vi "Main.vi"() -> ()   [LabVIEW 2020]
uses:
  <vilib>/userDefined/High Color/IMAQdx.ctl
  <vilib>/vision/driver/NI_Vision_Acquisition_Software.lvlib
panel:
  out "Status":bool
  in  "Off/On":bool caption="Start/Stop Vision"
  out "IMAQ Err":errorcluster
  out "Live view":T1(plugin-control)
  out "Python Error Out":errorcluster
  out "Camera Status":errorcluster
  in  "Exit program":bool
  in  "Camera Device":T2="cam0"
  # "Vision control panel"
  # "Camera configuration"
  # "Error section"
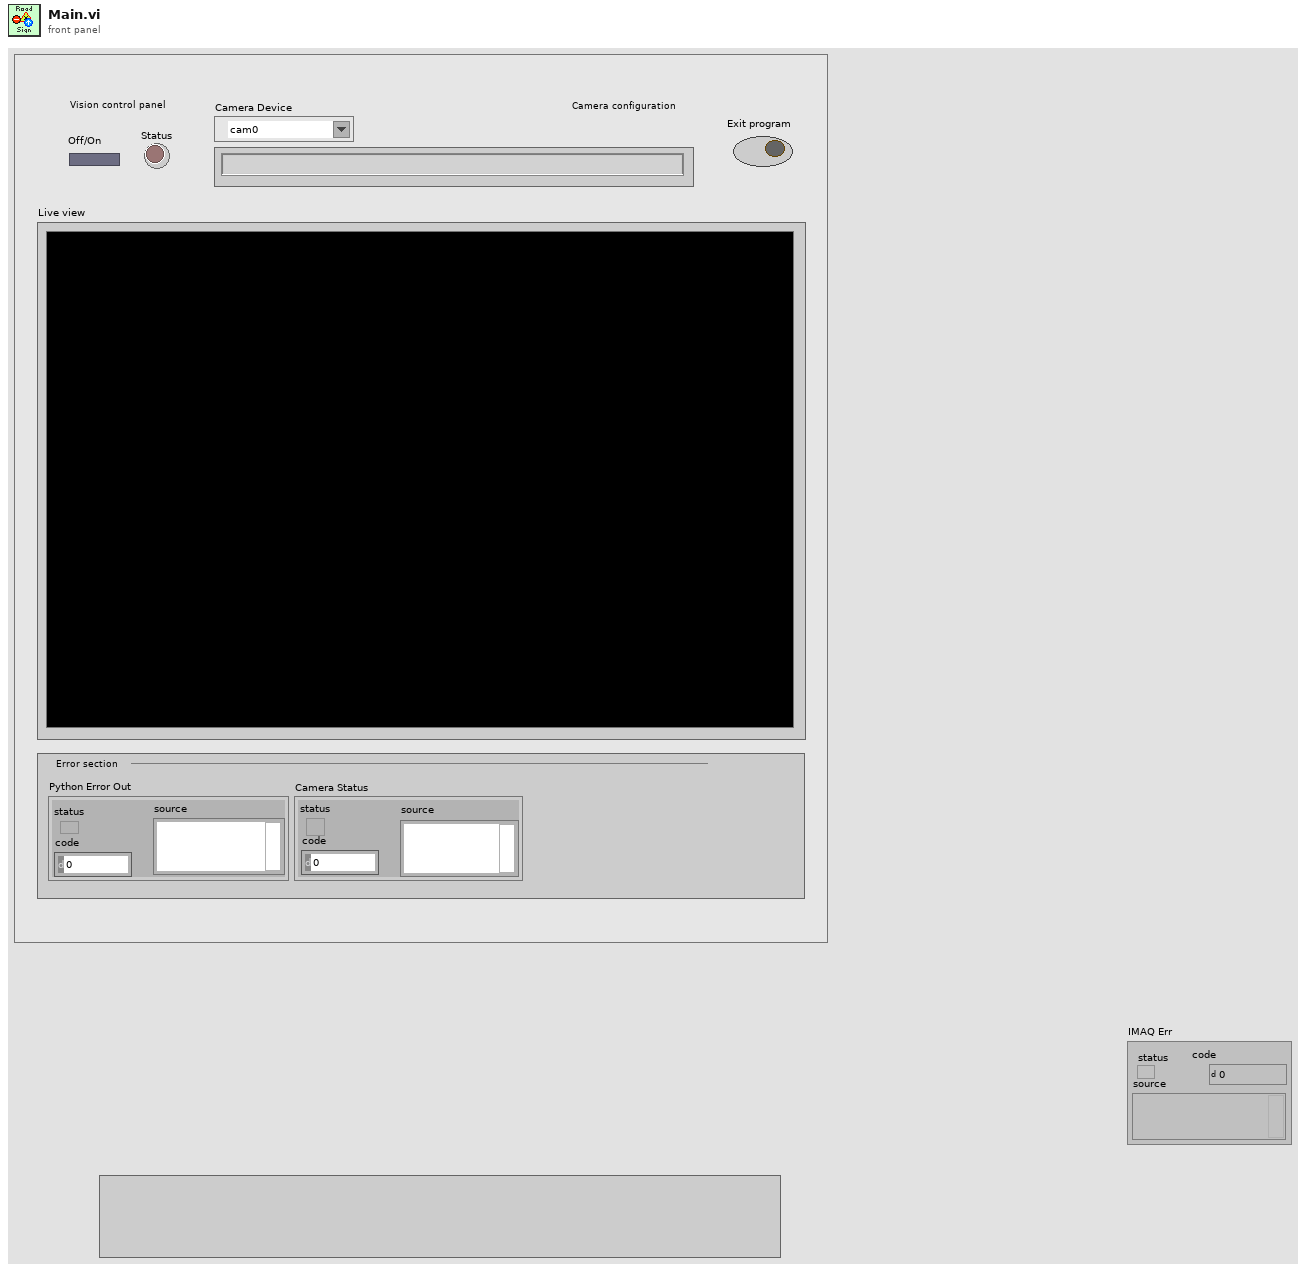
[diagram p1: front panel]
types:
  T1 = typedef "IMAQ Image.ctl" = refnum<image>
  T2 = typedef "IMAQdx.ctl" = refnum<k21>
  T3 = enum32{"Invalid", "Standard", "Closed", "Hidden", "Minimized", "Maximized"}
  T4 = enum32{"invalid app kind", "Development System", "Run Time System", "Student Edition", "Embedded LabVIEW", "Evaluation", "Custom"}
  T5 = cluster{"Core":cluster{"Current VI Reference":refnum<vi>, "Close Panel on Exit?":bool}, "Camera Device":T2}
  T6 = cluster{"Current VI Reference":refnum<vi>, "Close Panel on Exit?":bool}
  T7 = typedef "Image Type" = u32
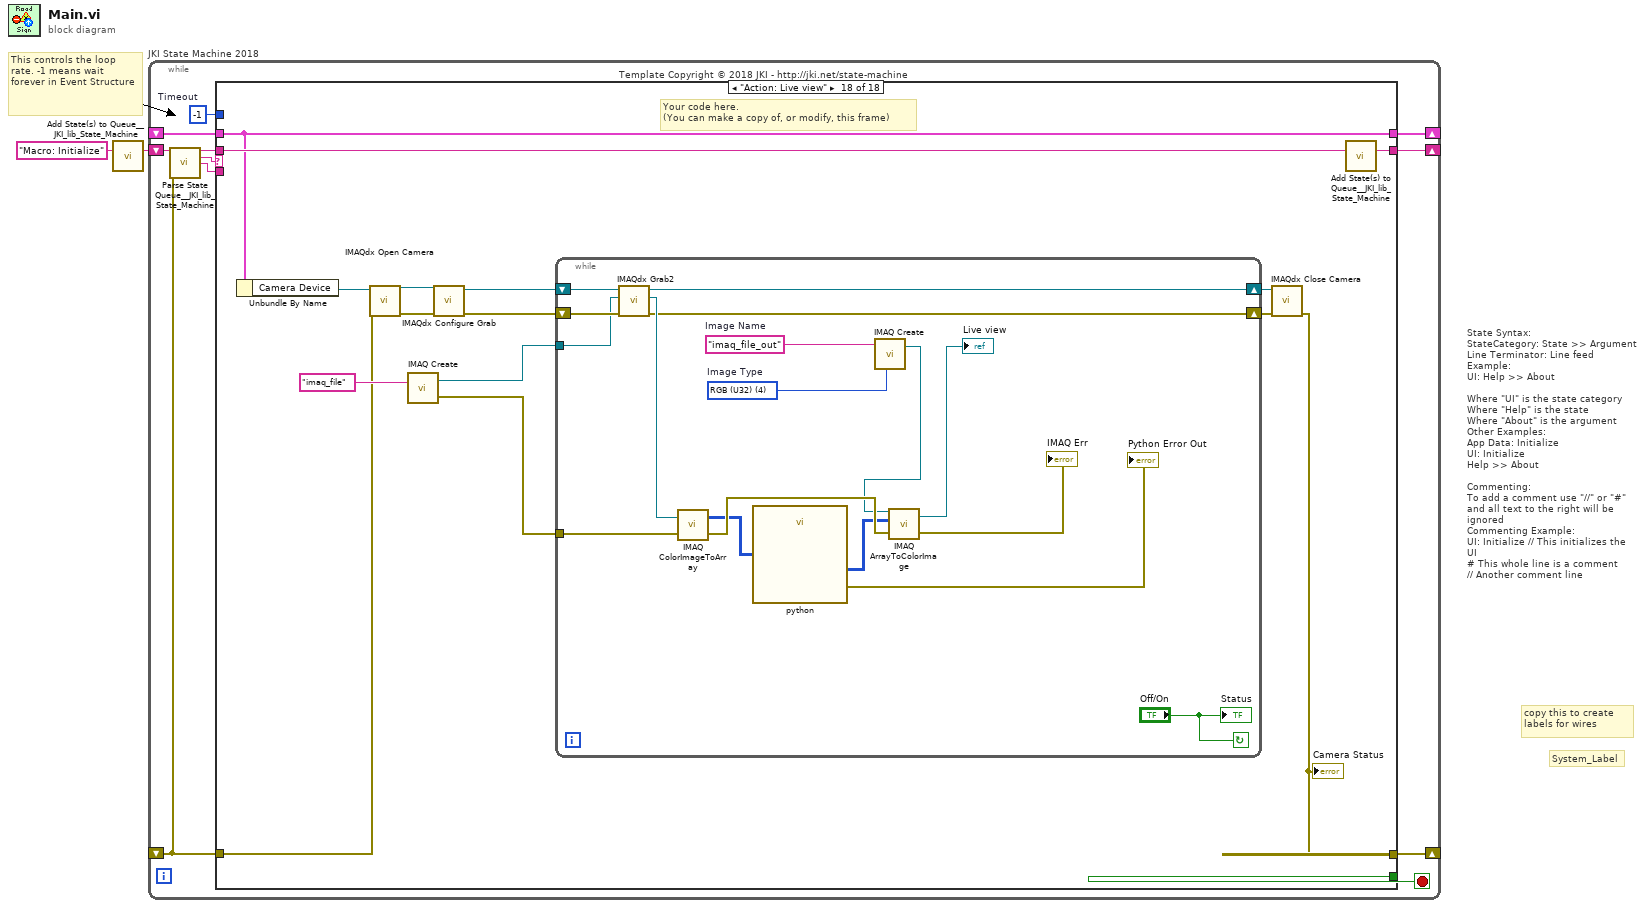
[diagram p0: block diagram]
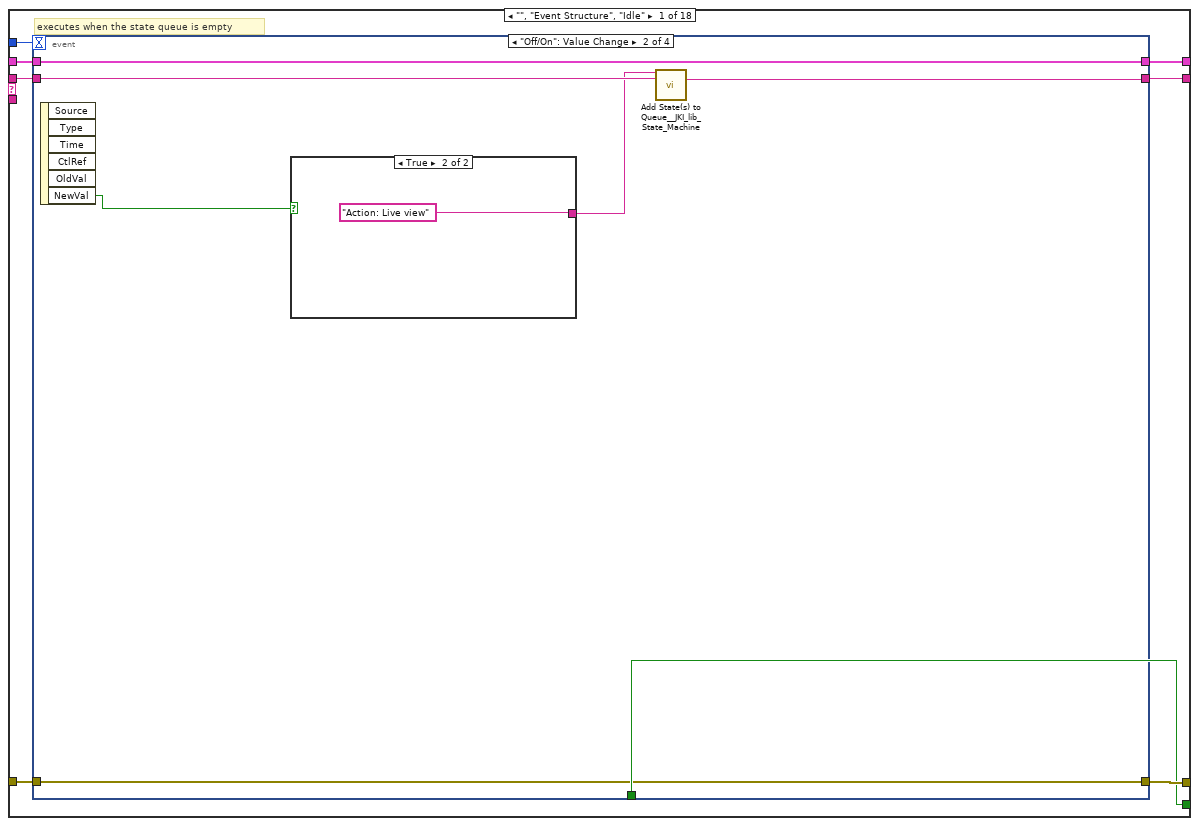
[diagram p2: hidden frame]
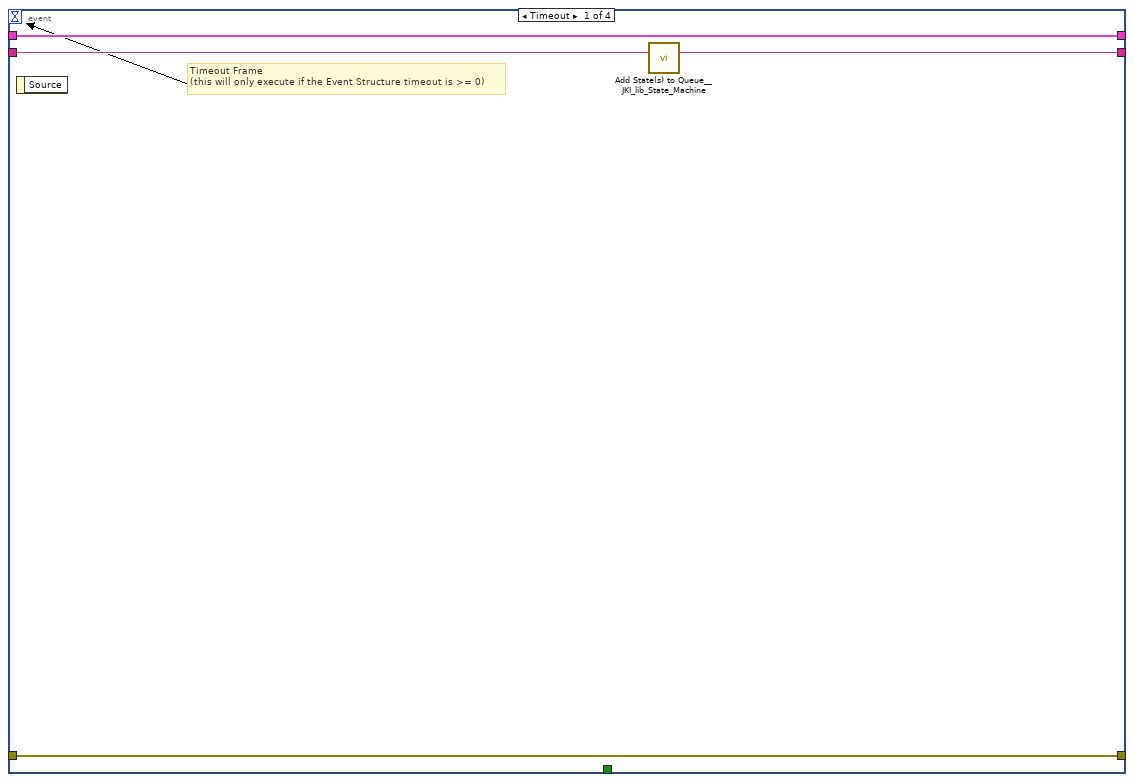
[diagram p3: hidden frame]
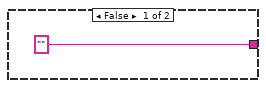
[diagram p4: hidden frame]
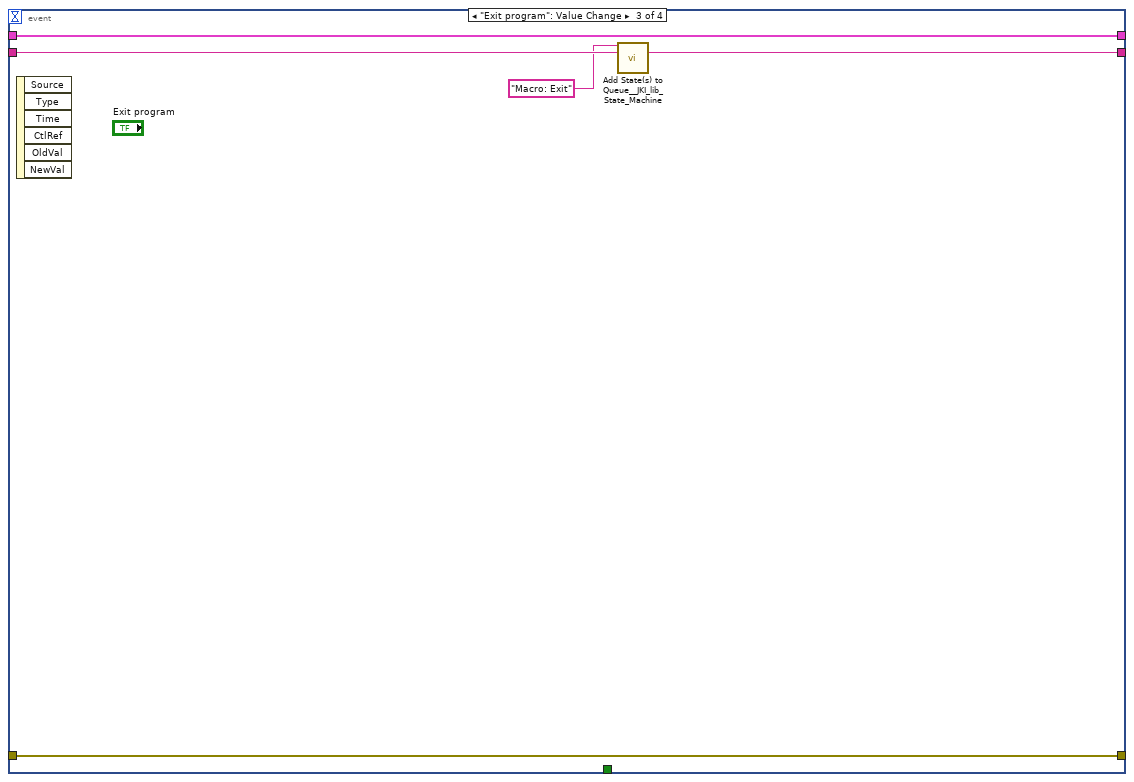
[diagram p5: hidden frame]
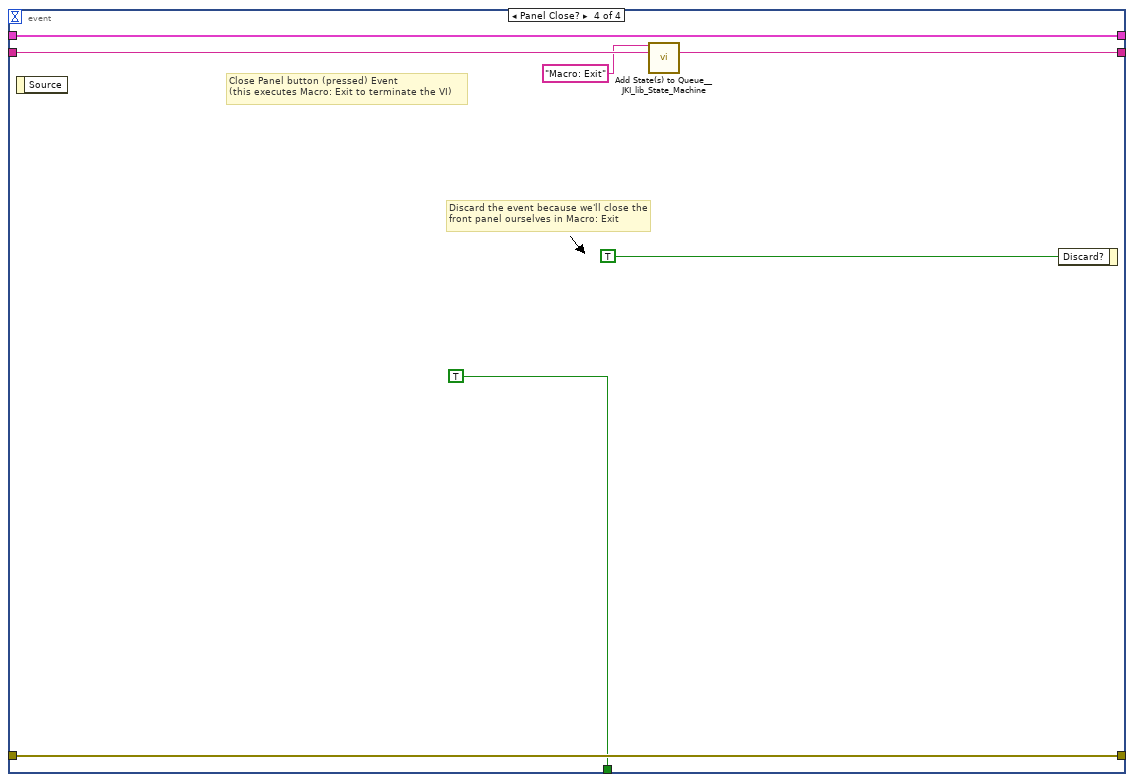
[diagram p6: hidden frame]
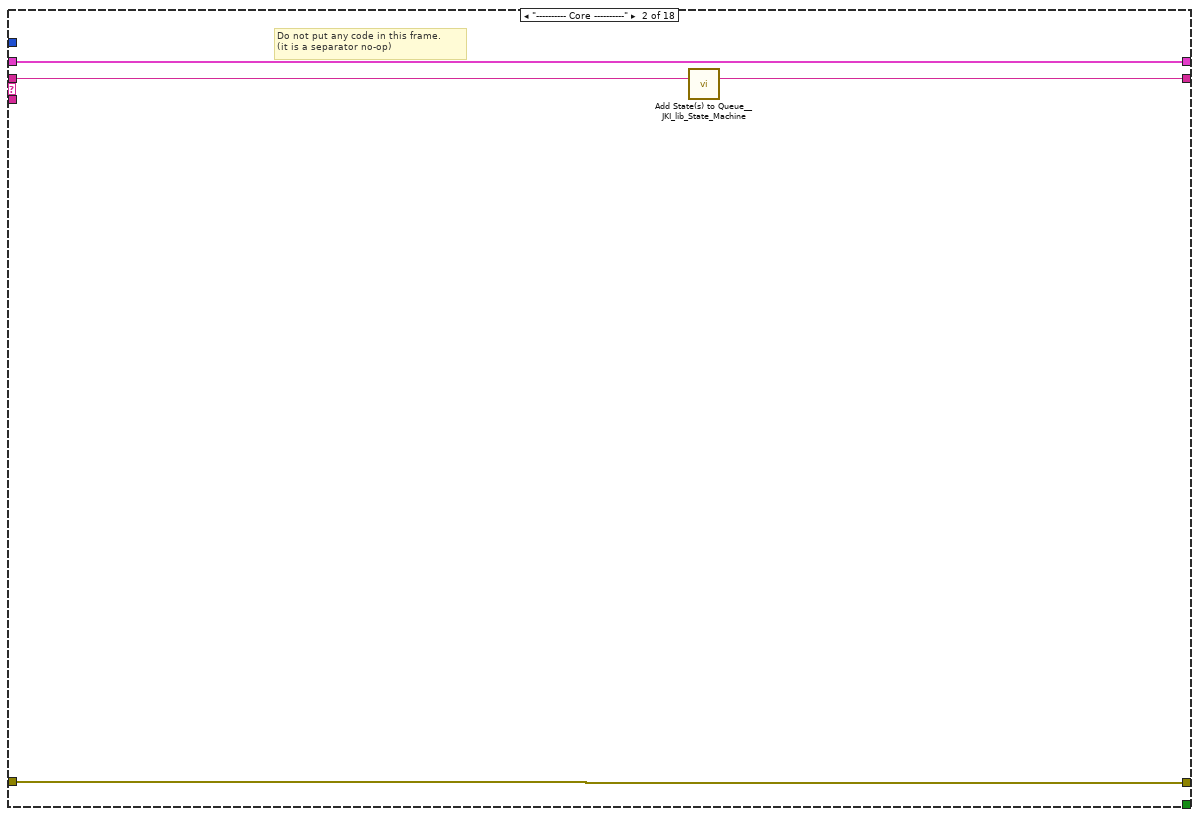
[diagram p7: hidden frame]
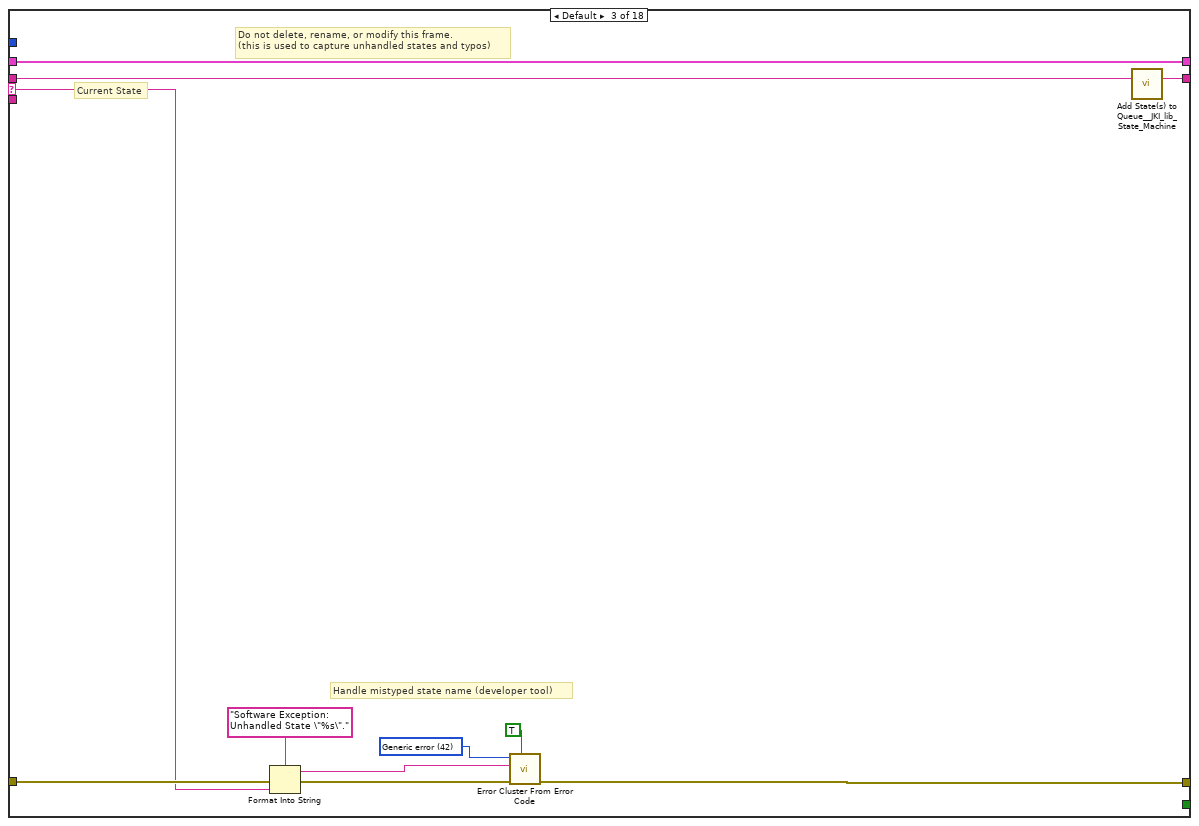
[diagram p8: hidden frame]
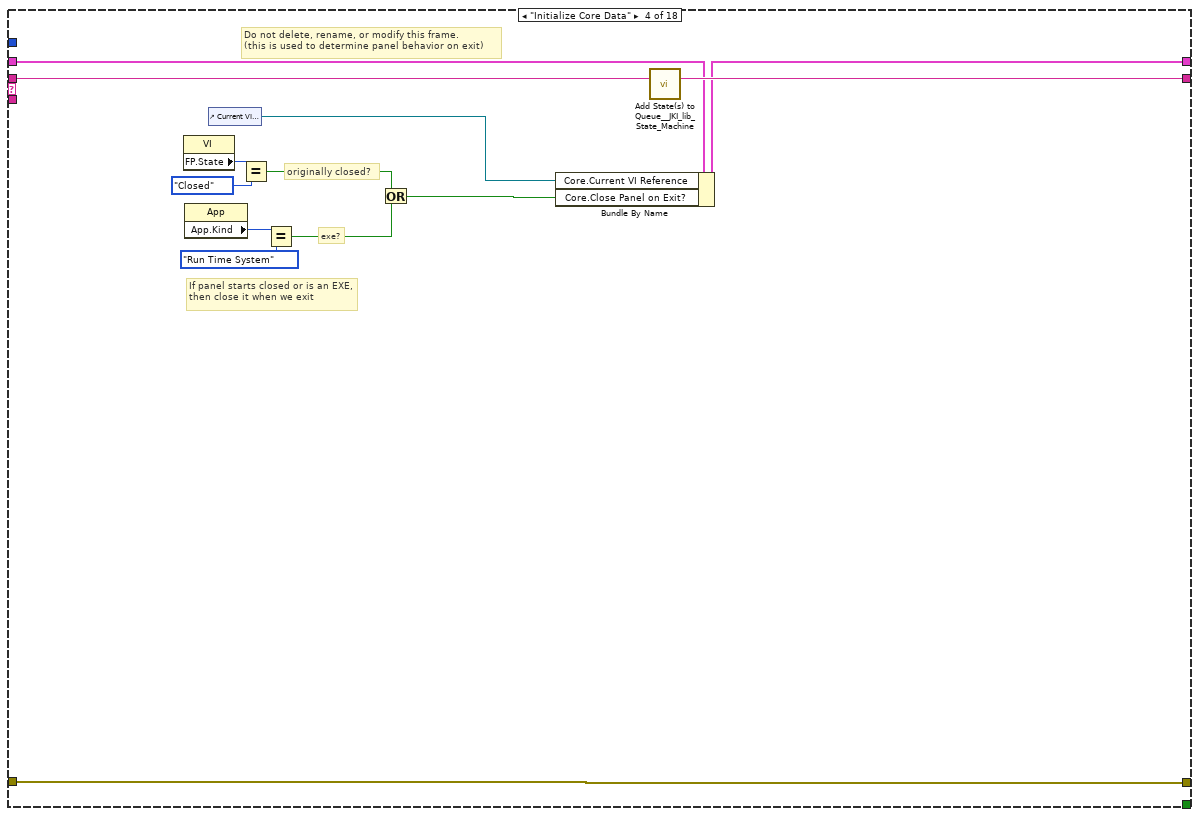
[diagram p9: hidden frame]
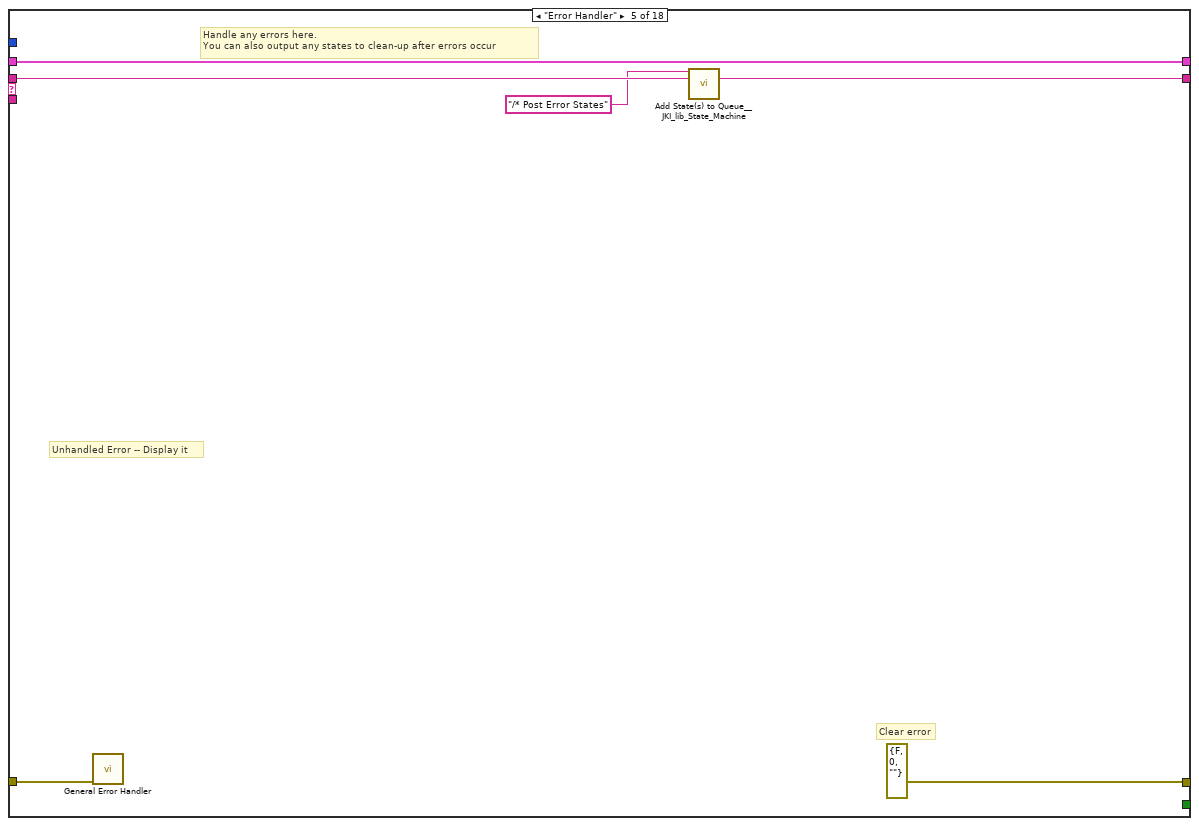
[diagram p10: hidden frame]
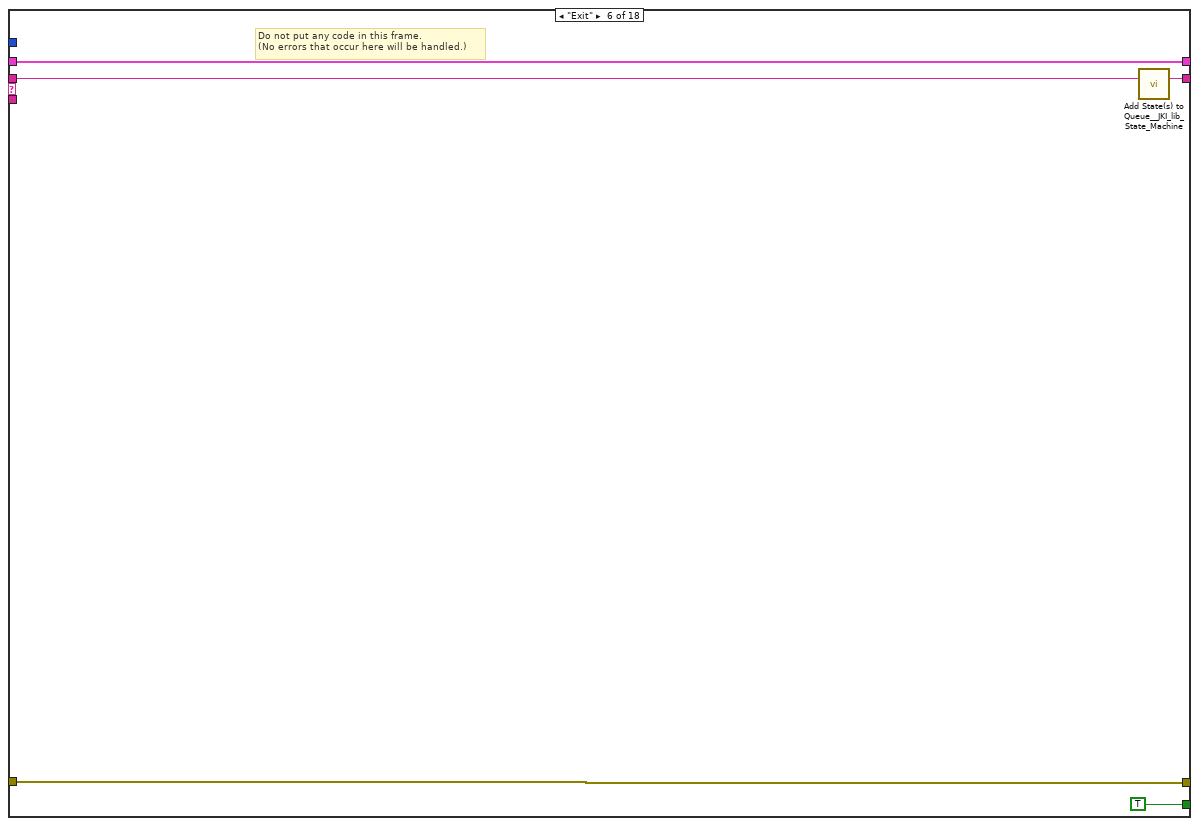
[diagram p11: hidden frame]
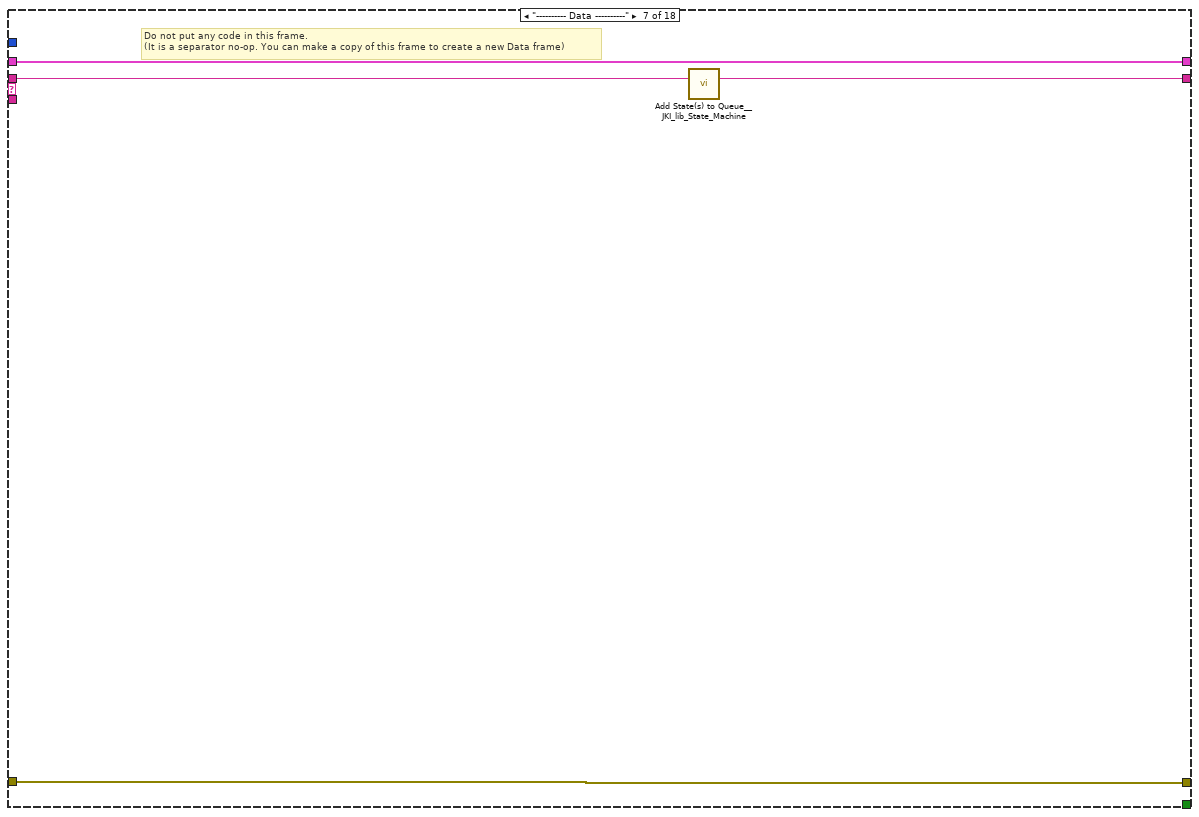
[diagram p12: hidden frame]
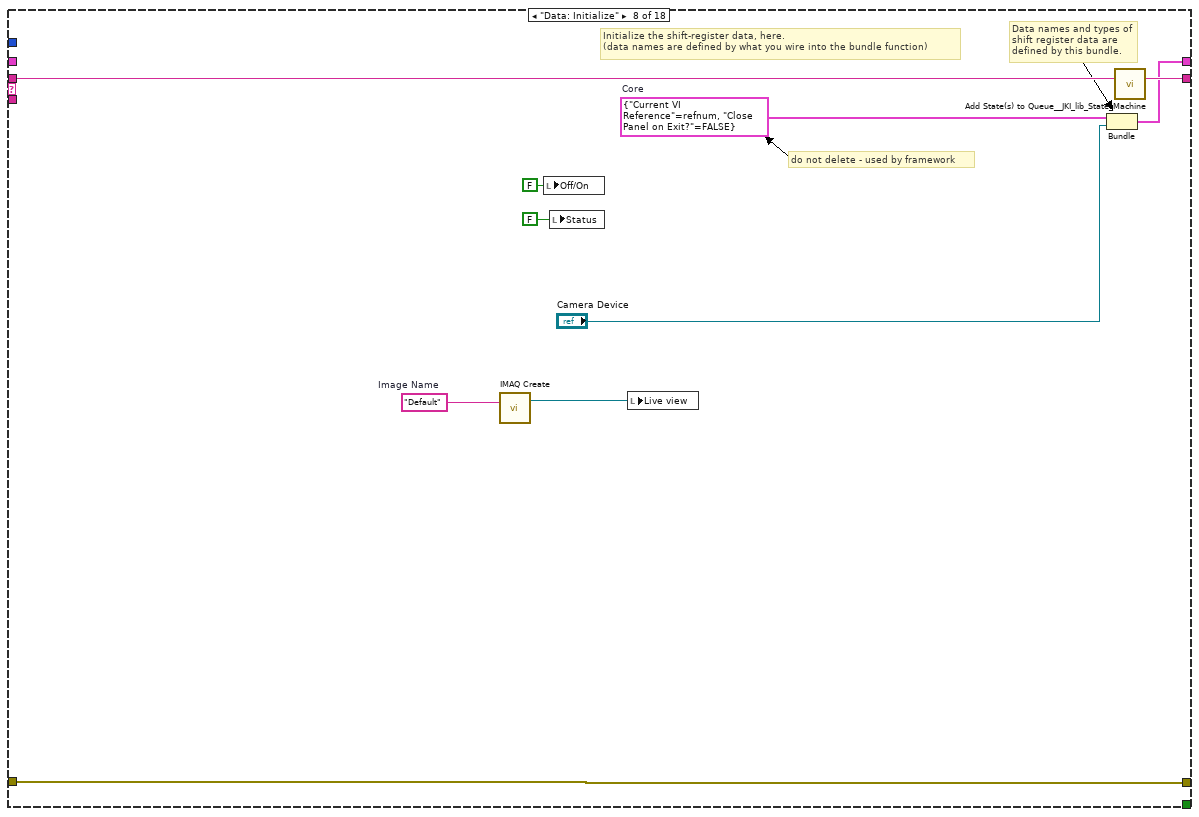
[diagram p13: hidden frame]
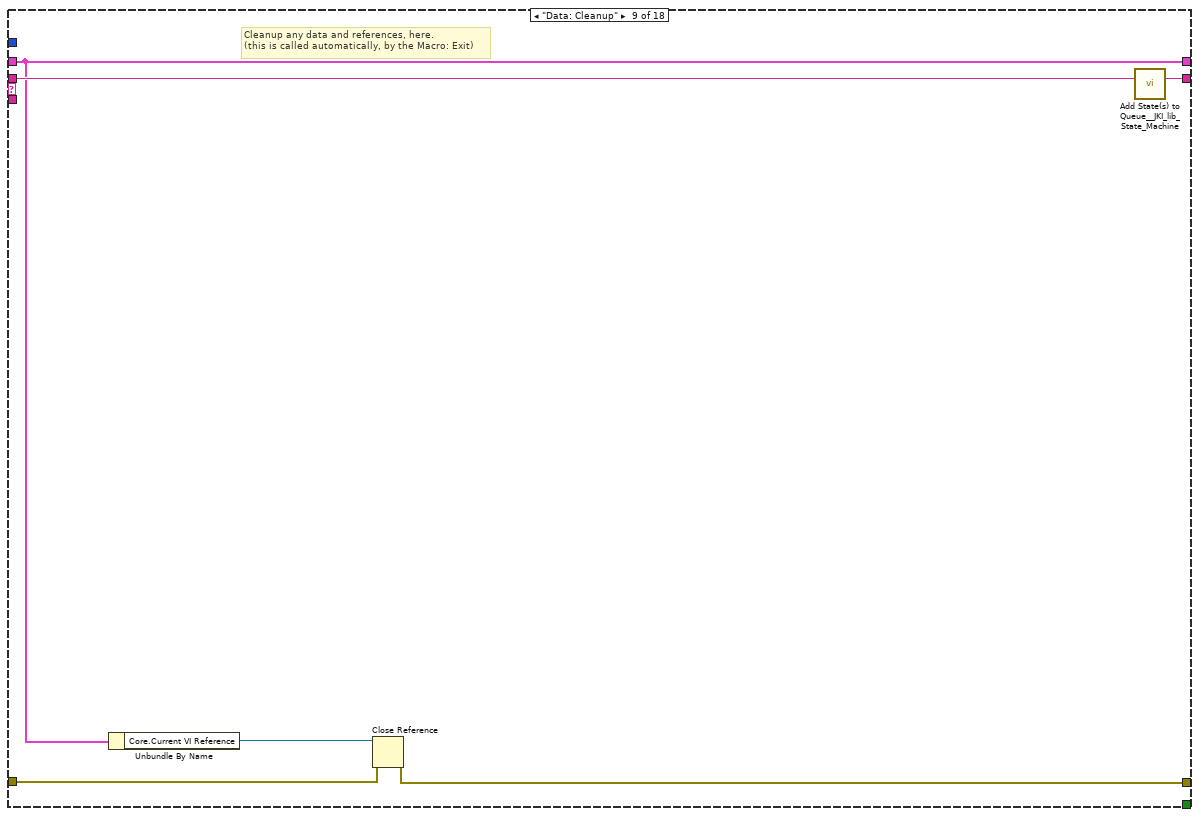
[diagram p14: hidden frame]
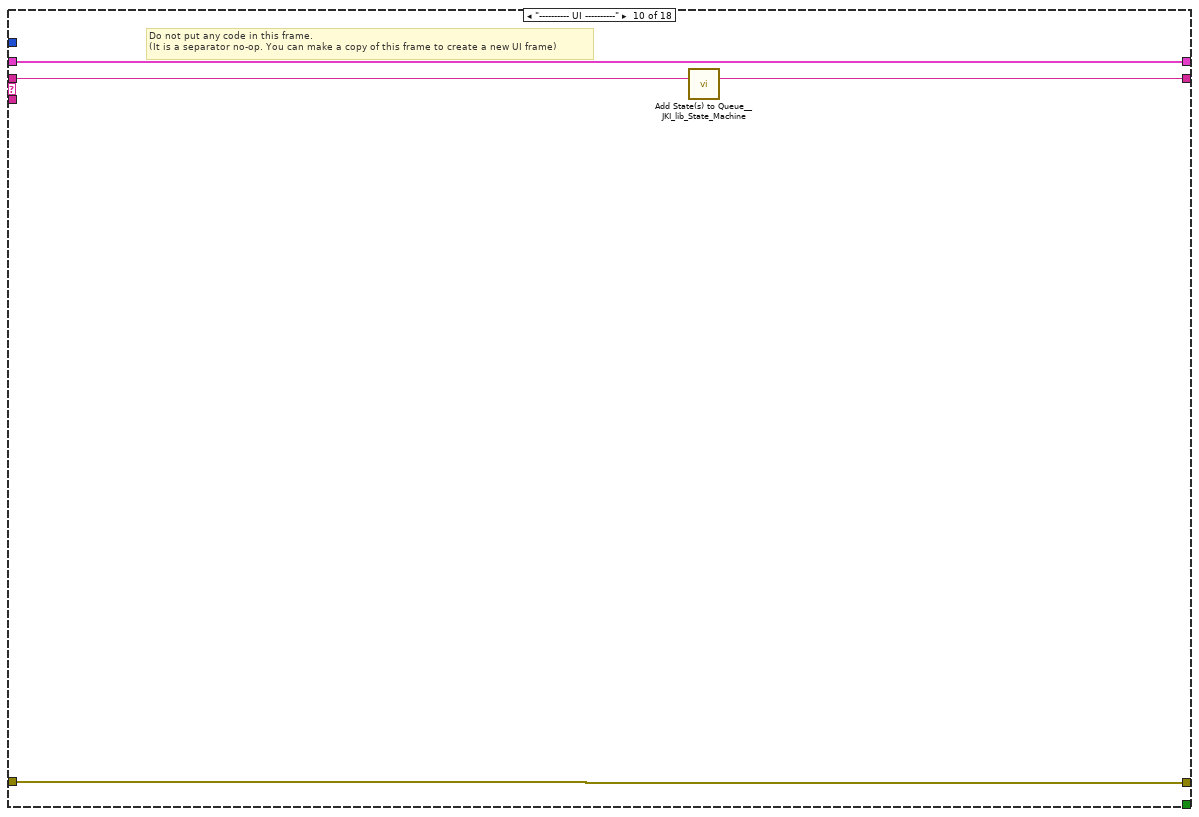
[diagram p15: hidden frame]
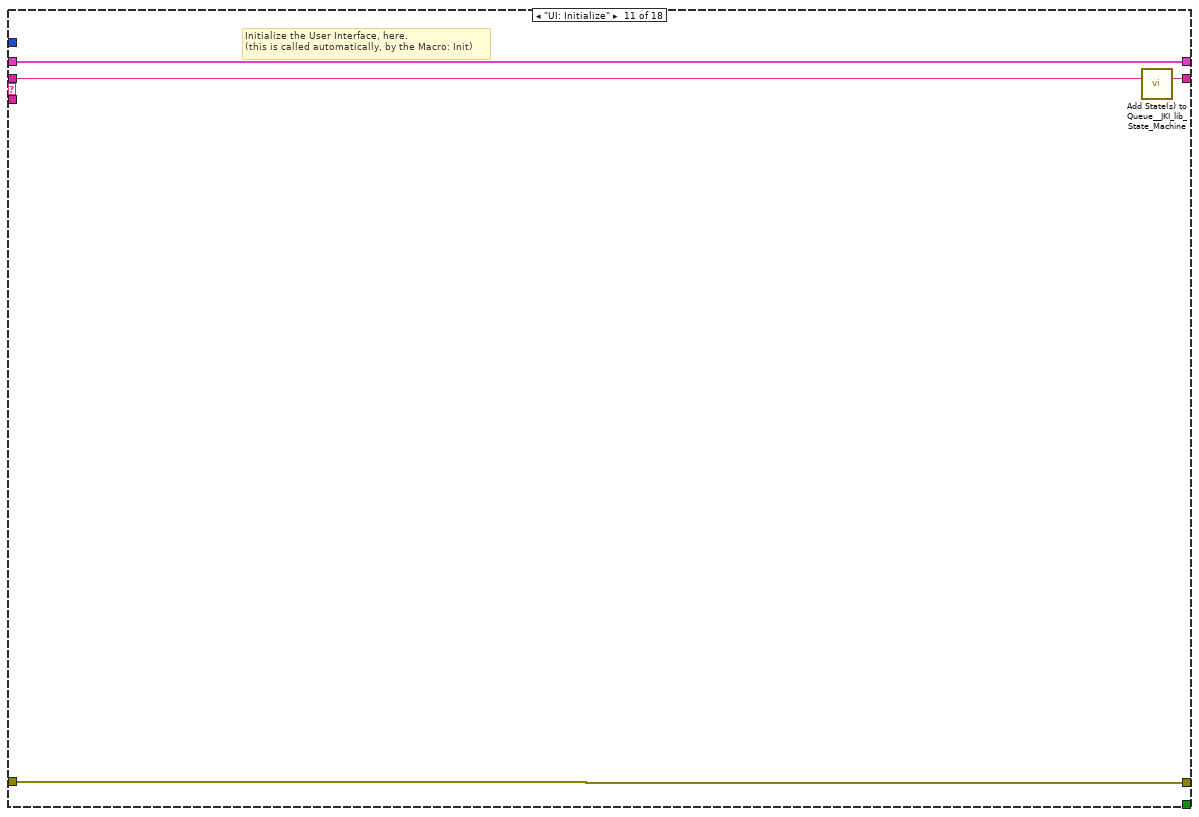
[diagram p16: hidden frame]
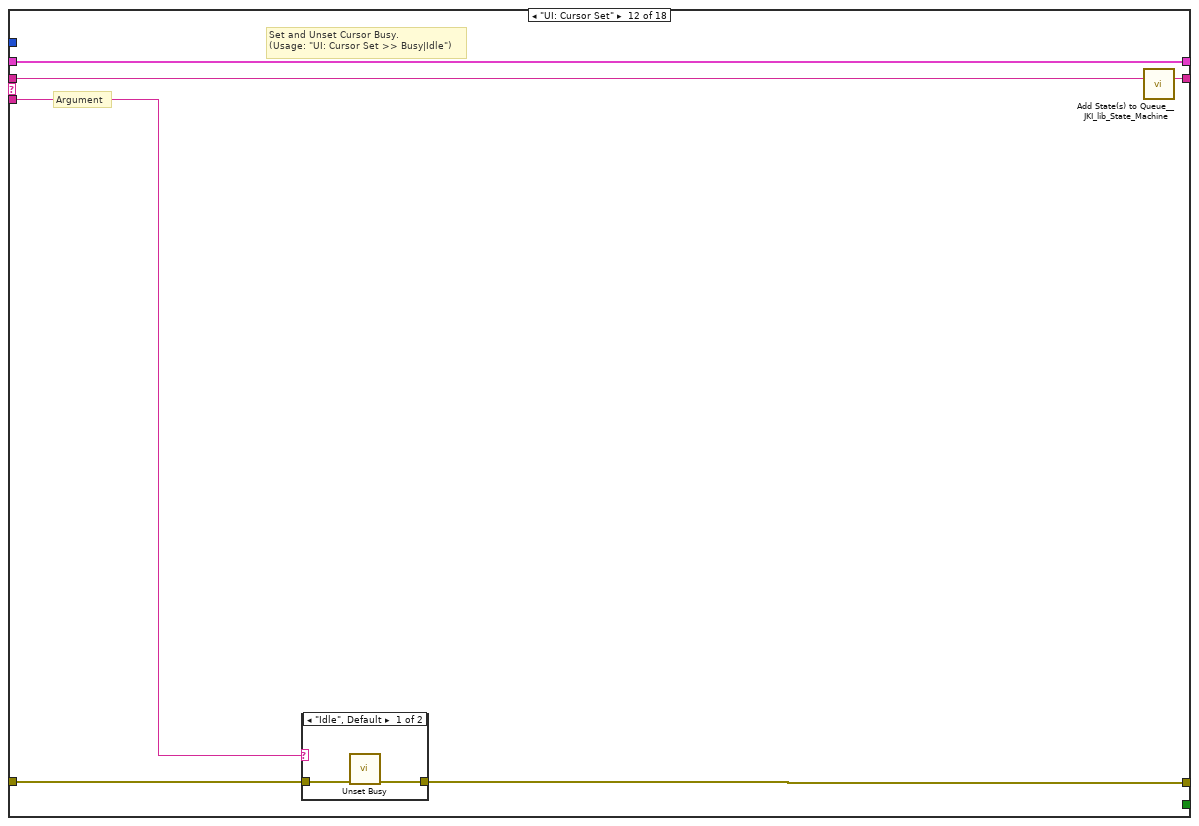
[diagram p17: hidden frame]
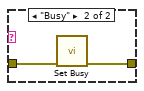
[diagram p18: hidden frame]
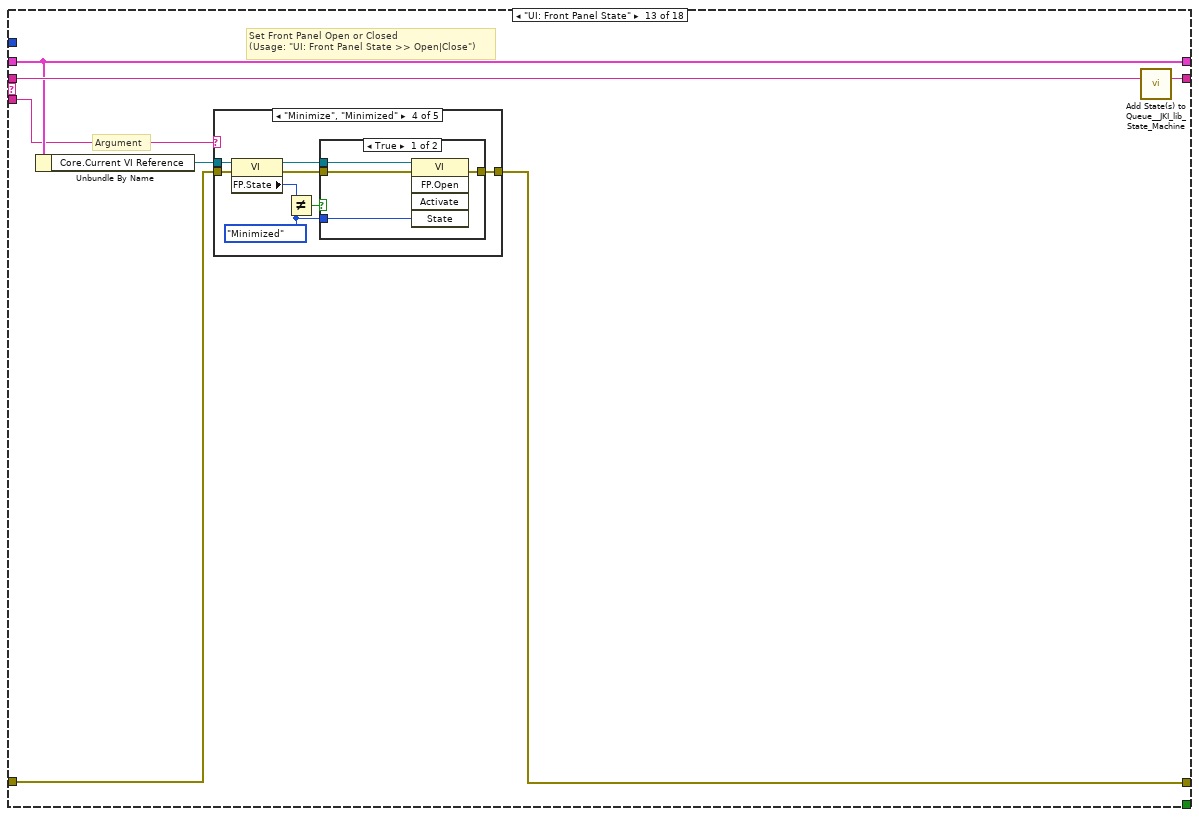
[diagram p19: hidden frame]
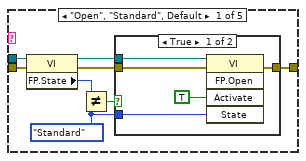
[diagram p20: hidden frame]
diagram:
  # "State Syntax:\nStateCategory: State >> Argument\nLine Terminator: Line feed\nExample:\nUI: Help >> About\n\nWhere \"UI\" is the state category\nWhere \"Help\" is the state\nWhere \"About\" is the argument\nOther Examples:\nApp Data: Initialize\nUI: Initialize\nHelp >> About\n\nCommenting:\nTo add a comment use \"//\" or \"#\" and all text to the right will be ignored\nCommenting Example:\nUI: Initialize // This initializes the UI\n# This whole line is a comment\n// Another comment line"
  # "copy this to create labels for wires"
  # "This controls the loop rate. -1 means wait forever in Event Structure"
  # "System_Label"
  n1 = call <vilib>:"Add State(s) to Queue__JKI_lib_State_Machine.vi"("State(s) in (\"\")"="Macro: Initialize") -> ("States Out"=w2:string)  [unwired: 14 in]
  n2 = while "JKI State Machine 2018" {
    shift-right: [w6] -> _
    shift-left: _ -> [w5]
    shift-right: [w9] -> _
    shift-left: _ -> [w3]
    shift-right: [w8] -> _
    shift-left: w2 -> [w10]
    stop <- w7 stop-if-true
    w4 = -1  # Timeout
    # "Template Copyright © 2018 JKI - http://jki.net/state-machine"
    n3 = call <vilib>:"Parse State Queue__JKI_lib_State_Machine.vi"("State Queue"=w10, "Error In (no error)"=w3) -> ("Remaining States"=w12:string, "Current State"=w13:string, "Arguments"=w11:string)  [unwired: 11 in]
    n4 = case shown="\"Action: Live view\"" w13 {
      selector: w13 -> [_ _ w50 _ _ _ _ _ _ _ _ _ _ _ _ _ _ _]
      tunnel: w12 -> [w21 w49 w54 w73 w79 w84 w88 w98 w104 w108 w112 w118 w129 w198 w203 w213 w217 w232]
      tunnel: w11 -> [_ _ _ _ _ _ _ _ _ _ _ w113 w123 _ _ _ _ _]
      tunnel: w5 -> [w19 w46 w52 w66 w76 w82 w85 _ w99 w105 w110 w116 w125 w195 w200 w210 w214 w228]
      tunnel: [w18 w47 w56 w70 errorcluster {"status"=FALSE, "code"=0, "source"=""} ("error out") w81 w86 w95 w100 w106 w109 w114 w126 w196 w201 w211 w215 w224] -> w9
      tunnel: w3 -> [w17 w47 w55 w70 w75 w81 w86 w95 w101 w106 w109 w115 w127 w196 w201 w211 w215 w225]
      tunnel: [w20 w48 w53 w72 w78 w83 w87 w97 w103 w107 w111 w117 w128 w197 w202 w212 w216 w231] -> w8
      tunnel: [w14 _ _ _ _ TRUE _ _ _ _ _ _ _ _ _ _ _ _] -> w7
      tunnel: [w16 w46 w52 w71 w76 w82 w85 w96 w99 w105 w110 w116 w125 w195 w200 w210 w214 w228] -> w6
      tunnel: w4 -> [w15 _ _ _ _ _ _ _ _ _ _ _ _ _ _ _ _ _]
      frame "", "Event Structure", "Idle" {
        # "executes when the state queue is empty"
        n5 = event shown="[1] \"Off/On\": Value Change" {
          selector: _ -> [_ _ _ _]
          dyn-events: _ -> [_ _ _ _]
          timeout: w15 -> [_ _ _ _]
          tunnel: w21 -> [w25 w28 w36 w45]
          tunnel: [w24 w29 w37 w44] -> w20
          tunnel: w19 -> [w22 w31 w38 w42]
          tunnel: [w23 w30 w34 w43] -> w18
          tunnel: w17 -> [w23 w30 w34 w43]
          tunnel: [w22 w31 w38 w42] -> w16
          tunnel: [_ _ _ TRUE] -> w14
          event Timeout {
            # "Timeout Frame\n(this will only execute if the Event Structure timeout is >= 0)"
            n6 = event-data() -> ()  [unwired: 1 in, 1 out]
            n7 = call <vilib>:"Add State(s) to Queue__JKI_lib_State_Machine.vi"("State(s) in (\"\")"=w25) -> ("States Out"=w24:string)  [unwired: 14 in]
          }
          event "Off/On": Value Change {
            n8 = event-data() -> ("NewVal"=w26:bool)  [unwired: 1 in, 5 out]
            n9 = case shown="True" w26 {
              tunnel: ["" "Action: Live view" ("State(s) in Front (\"\")")] -> w27
              frame False {
              }
              frame True {
              }
            }
            n10 = call <vilib>:"Add State(s) to Queue__JKI_lib_State_Machine.vi"("State(s) in Front (\"\")"=w27, "State(s) in (\"\")"=w28) -> ("States Out"=w29:string)  [unwired: 13 in]
          }
          event "Exit program": Value Change {
            n11 = event-data() -> ()  [unwired: 1 in, 6 out]
            n12 = call <vilib>:"Add State(s) to Queue__JKI_lib_State_Machine.vi"("State(s) in Front (\"\")"="Macro: Exit" ("State(s) in Front (\"\")"), "State(s) in (\"\")"=w36) -> ("States Out"=w37:string)  [unwired: 13 in]
          }
          event Panel Close? {
            # "Discard the event because we'll close the front panel ourselves in Macro: Exit"
            # "Close Panel button (pressed) Event\n(this executes Macro: Exit to terminate the VI)"
            n13 = event-data() -> ()  [unwired: 1 in, 1 out]
            n14 = call <vilib>:"Add State(s) to Queue__JKI_lib_State_Machine.vi"("State(s) in Front (\"\")"="Macro: Exit", "State(s) in (\"\")"=w45) -> ("States Out"=w44:string)  [unwired: 13 in]
            n15 = event-data("Discard?"=TRUE) -> ()  [unwired: 1 in, 1 out]
          }
        }
      }
      frame "---------- Core ----------" {
        # "Do not put any code in this frame.\n(it is a separator no-op)"
        n16 = call <vilib>:"Add State(s) to Queue__JKI_lib_State_Machine.vi"("State(s) in (\"\")"=w49) -> ("States Out"=w48:string)  [unwired: 14 in]
      }
      frame Default {
        w59 = 42 items=["No error", "Argument error", "Memory is full", "Out of zone", "End of file", "File already open", "Generic file I/O error", "File not found", "File permission error", "Disk is full", "Duplicate path", "Too many files open", "System feature not enabled", "Resource file not found", "Cannot add resource", "Resource not found", "Image not found", "Image memory error", "Pen does not exist", "Config type invalid", "Config token not found", "Config parse error", "Config memory error", "Bad external code format", "Bad external code offset", "External code not present", "Null window", "Destroy window error", "Null menu", "Print aborted", "Bad print record", "Print driver error", "Windows error during printing", "Memory error during printing", "Print dialog error", "Generic print error", "Invalid device refnum", "Device not found", "Device parameter error", "Device unit error", "Cannot open device", "Device call aborted", "Generic error", "Cancelled by user", "Object ID too low", "Object ID too high", "Object not in heap", "Unknown heap", "Unknown object (invalid DefProc)", "Unknown object (DefProc not in table)", "Message out of range", "Invalid (null) method", "Unknown message", "Manager call not supported", "Bad address", "Network operation in progress", "Network operation timed out", "Connection is busy", "Network attribute not supported", "Network error", "Address in use", "System out of memory", "Connection aborted", "Connection refused", "Not connected", "Already connected", "Connection closed", "Initialization error (interapplication manager)", "Bad occurrence", "Wait on unbound occurrence handler", "Occurrence queue overflow", "Datalog type conflict", "Unused", "Unrecognized type (interapplication manager)", "Memory corrupt", "Failed to make temporary DLL", "Old CIN version", "Drag socket not found", "Failed to load drop-object", "Failed to register OLE object", "Failed to release OLE object", "Format specifier type mismatch", "Unknown format specifier", "Too few format specifiers", "Too many format specifiers", "Scan failed", "Newer CIN version", "Error converting to variant", "Runtime menu error", "Password tampered", "Variant attribute not found", "Incompatible variant data type", "Event data is not available", "Event Store is not present", "Occurrence is not found", "Event Queue is not created", "Event info is not available", "Refnum passed is NULL", "Error retrieving Class GUID", "Error retrieving CoClass GUID", "Error retrieving TypeLib GUID.", "Bad built application magic bytes.", "Specific driver is different from the specific driver associated with the Logical Name.", "There is no session opened to the class driver.", "Max Error", "MAX - Error with config objects", "MAX - Error loading configuration", "MAX - Group not supported"]
        # "Current State"
        # "Do not delete, rename, or modify this frame.\n(this is used to capture unhandled states and typos)"
        # "Handle mistyped state name (developer tool)"
        n17 = Format Into String(format string="Software Exception: Unhandled State \"%s\"." ("message"), error in=w55, w50) -> (resulting string=w58:string, error out=w57:errorcluster)  [unwired: 1 in]
        n18 = call <vilib>:"Error Cluster From Error Code.vi"("show call chain? (False)"=TRUE, "error in (no error)"=w57, "error message (\"\")"=w58, "error code (0)"=w59) -> ("error out"=w56:errorcluster)  [unwired: 5 in]
        n19 = call <vilib>:"Add State(s) to Queue__JKI_lib_State_Machine.vi"("State(s) in (\"\")"=w54) -> ("States Out"=w53:string)  [unwired: 14 in]
      }
      frame "Initialize Core Data" {
        # "Do not delete, rename, or modify this frame.\n(this is used to determine panel behavior on exit)"
        # "originally closed?"
        # "exe?"
        # "If panel starts closed or is an EXE, then close it when we exit"
        n20 = property class="VI"() -> ("FP.State"=w63:T3)  [unwired: 2 in, 2 out]
        n21 = property class="App"() -> ("App.Kind"=w69:T4)  [unwired: 2 in, 2 out]
        n22 = control-ref of="Current VI Reference"() -> (w64:refnum<vi>)
        n23 = Equal?(x=w63, y=T3."Closed" ("Front Panel Window:State")) -> (x = y?=w61:bool)
        n24 = Equal?(x=w69, y=T4."Run Time System" ("Application:Kind")) -> (x = y?=w67:bool)
        n25 = Or(x=w61, y=w67) -> (x .or. y?=w65:bool)
        n26 = Bundle By Name(cluster=w66, "Core.Current VI Reference"=w64, "Core.Close Panel on Exit?"=w65) -> (w71:T5)
        n27 = call <vilib>:"Add State(s) to Queue__JKI_lib_State_Machine.vi"("State(s) in (\"\")"=w73) -> ("States Out"=w72:string)  [unwired: 14 in]
      }
      frame "Error Handler" {
        # "Unhandled Error -- Display it"
        # "Handle any errors here.\nYou can also output any states to clean-up after errors occur"
        # "Clear error"
        n28 = call <vilib>:"General Error Handler.vi"("error in (no error)"=w75) -> ()  [unwired: 10 in, 5 out]
        n29 = call <vilib>:"Add State(s) to Queue__JKI_lib_State_Machine.vi"("State(s) in Front (\"\")"="/* Post Error States", "State(s) in (\"\")"=w79) -> ("States Out"=w78:string)  [unwired: 13 in]
      }
      frame "Exit" {
        # "Do not put any code in this frame.\n(No errors that occur here will be handled.)"
        n30 = call <vilib>:"Add State(s) to Queue__JKI_lib_State_Machine.vi"("State(s) in (\"\")"=w84) -> ("States Out"=w83:string)  [unwired: 14 in]
      }
      frame "---------- Data ----------" {
        # "Do not put any code in this frame.\n(It is a separator no-op. You can make a copy of this frame to create a new Data frame)"
        n31 = call <vilib>:"Add State(s) to Queue__JKI_lib_State_Machine.vi"("State(s) in (\"\")"=w88) -> ("States Out"=w87:string)  [unwired: 14 in]
      }
      frame "Data: Initialize" {
        w90 = "Default"  # Image Name
        w94 = T6 {"Current VI Reference"=refnum, "Close Panel on Exit?"=FALSE}  # Core
        # "do not delete - used by framework"
        # "Data names and types of shift register data are defined by this bundle."
        # "Initialize the shift-register data, here.\n(data names are defined by what you wire into the bundle function)"
        n32 = call "IMAQ Create"("Image Name"=w90) -> ("New Image"=w89:T1)  [unwired: 4 in, 1 out]
        n33 = local write "Off/On"(FALSE ("Status")) -> ()
        n34 = local write "Status"(FALSE ("Off/On")) -> ()
        n35 = local write "Live view"(w89) -> ()
        n36 = Bundle("Core"=w94, "Camera Device"="Camera Device") -> (w96:T5)  [unwired: 1 in]
        n37 = call <vilib>:"Add State(s) to Queue__JKI_lib_State_Machine.vi"("State(s) in (\"\")"=w98) -> ("States Out"=w97:string)  [unwired: 14 in]
      }
      frame "Data: Cleanup" {
        # "Cleanup any data and references, here.\n(this is called automatically, by the Macro: Exit)"
        n38 = Unbundle By Name(w99) -> ("Core.Current VI Reference"=w102:refnum<vi>)
        n39 = Close Reference(reference=w102, error in (no error)=w101) -> (error out=w100:errorcluster)
        n40 = call <vilib>:"Add State(s) to Queue__JKI_lib_State_Machine.vi"("State(s) in (\"\")"=w104) -> ("States Out"=w103:string)  [unwired: 14 in]
      }
      frame "---------- UI ----------" {
        # "Do not put any code in this frame.\n(It is a separator no-op. You can make a copy of this frame to create a new UI frame)"
        n41 = call <vilib>:"Add State(s) to Queue__JKI_lib_State_Machine.vi"("State(s) in (\"\")"=w108) -> ("States Out"=w107:string)  [unwired: 14 in]
      }
      frame "UI: Initialize" {
        # "Initialize the User Interface, here.\n(this is called automatically, by the Macro: Init)"
        n42 = call <vilib>:"Add State(s) to Queue__JKI_lib_State_Machine.vi"("State(s) in (\"\")"=w112) -> ("States Out"=w111:string)  [unwired: 14 in]
      }
      frame "UI: Cursor Set" {
        # "Argument"
        # "Set and Unset Cursor Busy.\n(Usage: \"UI: Cursor Set >> Busy|Idle\")"
        n43 = case shown="\"Idle\", Default" w113 {
          tunnel: w115 -> [w120 w122]
          tunnel: [w119 w121] -> w114
          frame "Idle", Default {
            n44 = call <vilib>:"Unset Busy.vi"("error in (no error)"=w120) -> ("error out"=w119:errorcluster)  [unwired: 10 in]
          }
          frame "Busy" {
            n45 = call <vilib>:"Set Busy.vi"("error in (no error)"=w122) -> ("error out"=w121:errorcluster)  [unwired: 9 in, 1 out]
          }
        }
        n46 = call <vilib>:"Add State(s) to Queue__JKI_lib_State_Machine.vi"("State(s) in (\"\")"=w118) -> ("States Out"=w117:string)  [unwired: 14 in]
      }
      frame "UI: Front Panel State" {
        # "Argument"
        # "Set Front Panel Open or Closed\n(Usage: \"UI: Front Panel State >> Open|Close\")"
        n47 = Unbundle By Name(w125) -> ("Core.Current VI Reference"=w124:refnum<vi>)
        n48 = case shown="\"Minimize\", \"Minimized\"" w123 {
          tunnel: w127 -> [w135 w150 w161 w174 w187]
          tunnel: [w137 w151 w163 w176 w189] -> w126
          tunnel: w124 -> [w136 w148 w162 w175 w188]
          frame "Open", "Standard", Default {
            w130 = T3."Standard" ("State")
            n49 = property class="VI"(reference=w136, error in=w135) -> (reference out=w133:refnum<vi>, error out=w134:errorcluster, "FP.State"=w132:T3)
            n50 = Not Equal?(x=w132, y=w130) -> (x != y?=w131:bool)
            n51 = case shown="True" w131 {
              tunnel: [w141 w143] -> w137
              tunnel: w134 -> [w140 w143]
              tunnel: w133 -> [w139 _]
              tunnel: w130 -> [w138 _]
              frame True {
                n52 = invoke class="VI" method="FP.Open"(reference=w139, error in=w140, "Activate"=TRUE, "State"=w138) -> (error out=w141:errorcluster)  [unwired: 1 in, 4 out]
              }
              frame False {
              }
            }
          }
          frame "Close", "Closed" {
            n53 = property class="VI"(reference=w148, error in=w150) -> (reference out=w147:refnum<vi>, error out=w149:errorcluster, "FP.State"=w145:T3)
            n54 = Not Equal?(x=w145, y=T3."Closed" ("Front Panel Window:State")) -> (x != y?=w144:bool)
            n55 = case shown="True" w144 {
              tunnel: [w152 w155] -> w151
              tunnel: w149 -> [w152 w154]
              tunnel: w147 -> [_ w153]
              frame False {
              }
              frame True {
                n56 = invoke class="VI" method="FP.Close"(reference=w153, error in=w154) -> (error out=w155:errorcluster)  [unwired: 1 in, 2 out]
              }
            }
          }
          frame "Hidden", "Hide" {
            w156 = T3."Hidden" ("State")
            n57 = property class="VI"(reference=w162, error in=w161) -> (reference out=w159:refnum<vi>, error out=w160:errorcluster, "FP.State"=w158:T3)
            n58 = Not Equal?(x=w158, y=w156) -> (x != y?=w157:bool)
            n59 = case shown="True" w157 {
              tunnel: [w167 w168] -> w163
              tunnel: w160 -> [w166 w168]
              tunnel: w159 -> [w165 _]
              tunnel: w156 -> [w164 _]
              frame True {
                n60 = invoke class="VI" method="FP.Open"(reference=w165, error in=w166, "State"=w164) -> (error out=w167:errorcluster)  [unwired: 2 in, 4 out]
              }
              frame False {
              }
            }
          }
          frame "Minimize", "Minimized" {
            w169 = T3."Minimized" ("State")
            n61 = property class="VI"(reference=w175, error in=w174) -> (reference out=w172:refnum<vi>, error out=w173:errorcluster, "FP.State"=w171:T3)
            n62 = Not Equal?(x=w171, y=w169) -> (x != y?=w170:bool)
            n63 = case shown="True" w170 {
              tunnel: [w180 w181] -> w176
              tunnel: w173 -> [w179 w181]
              tunnel: w172 -> [w178 _]
              tunnel: w169 -> [w177 _]
              frame True {
                n64 = invoke class="VI" method="FP.Open"(reference=w178, error in=w179, "State"=w177) -> (error out=w180:errorcluster)  [unwired: 2 in, 4 out]
              }
              frame False {
              }
            }
          }
          frame "Maximize", "Maximized" {
            w182 = T3."Maximized" ("State")
            n65 = property class="VI"(reference=w188, error in=w187) -> (reference out=w185:refnum<vi>, error out=w186:errorcluster, "FP.State"=w184:T3)
            n66 = Not Equal?(x=w184, y=w182) -> (x != y?=w183:bool)
            n67 = case shown="True" w183 {
              tunnel: [w193 w194] -> w189
              tunnel: w186 -> [w192 w194]
              tunnel: w185 -> [w191 _]
              tunnel: w182 -> [w190 _]
              frame True {
                n68 = invoke class="VI" method="FP.Open"(reference=w191, error in=w192, "State"=w190) -> (error out=w193:errorcluster)  [unwired: 2 in, 4 out]
              }
              frame False {
              }
            }
          }
        }
        n69 = call <vilib>:"Add State(s) to Queue__JKI_lib_State_Machine.vi"("State(s) in (\"\")"=w129) -> ("States Out"=w128:string)  [unwired: 14 in]
      }
      frame "---------- Macro ----------" {
        # "Do not put any code in this frame.\n(It is a separator no-op. You can make a copy of this frame to create a new Macro frame)"
        n70 = call <vilib>:"Add State(s) to Queue__JKI_lib_State_Machine.vi"("State(s) in (\"\")"=w198) -> ("States Out"=w197:string)  [unwired: 14 in]
      }
      frame "Macro: Initialize" {
        w199 = "Data: Initialize\nInitialize Core Data\nUI: Initialize\nUI: Front Panel State >> Open"  # Data: Initialize Initialize Core Data UI: Initialize UI: Front Panel State >> Open
        # "Initialization Macro\n(This is called once, when the VI starts)"
        n71 = call <vilib>:"Add State(s) to Queue__JKI_lib_State_Machine.vi"("State(s) in Front (\"\")"=w199, "State(s) in (\"\")"=w203) -> ("States Out"=w202:string)  [unwired: 13 in]
      }
      frame "Macro: Exit" {
        # "Exit Macro\n(This is called once, when the VI exits)"
        n72 = Unbundle By Name(w210) -> ("Core.Close Panel on Exit?"=w209:bool)
        n73 = Select(t="UI: Front Panel State >> Close", s=w209, f="") -> (s? t:f=w206:string)
        n74 = call <vilib>:"Add State(s) to Queue__JKI_lib_State_Machine.vi"("State(s) in (\"\")"=w206, "State(s) at Back (\"\")"="Data: Cleanup\nExit") -> ("States Out"=w204:string)  [unwired: 13 in]
        n75 = call <vilib>:"Add State(s) to Queue__JKI_lib_State_Machine.vi"("State(s) in Front (\"\")"=w204, "State(s) in (\"\")"=w213) -> ("States Out"=w212:string)  [unwired: 13 in]
      }
      frame "---------- Action ----------" {
        # "Template Separator\n(You can make a copy of, or modify, this frame)"
        n76 = call <vilib>:"Add State(s) to Queue__JKI_lib_State_Machine.vi"("State(s) in (\"\")"=w217) -> ("States Out"=w216:string)  [unwired: 14 in]
      }
      frame "Action: Live view" {
        # "Your code here.\n(You can make a copy of, or modify, this frame)"
        n77 = Unbundle By Name(w228) -> ("Camera Device"=w227:T2)
        n78 = call <vilib>:"IMAQdx Open Camera.vi"("error in"=w225, "Session In"=w227) -> ("error out"=w226:errorcluster, "Session Out"=w230:T2)  [unwired: 8 in]
        n79 = call "IMAQ Create"("Image Name"="imaq_file") -> ("New Image"=w221:T1, "error out"=w223:errorcluster)  [unwired: 4 in]
        n80 = call <vilib>:"IMAQdx Configure Grab.vi"("error in"=w226, "Session In"=w230) -> ("error out"=w222:errorcluster, "Session Out"=w220:T2)  [unwired: 8 in]
        n81 = while {
          tunnel: w223 -> [w242]
          tunnel: w221 -> [w240]
          shift-right: [w234] -> w219
          shift-left: w222 -> [w241]
          shift-right: [w236] -> w218
          shift-left: w220 -> [w239]
          stop <- "Off/On" continue-if-true
          w248 = T7 4 items=["Grayscale (U8)", "Grayscale (I16)", "Grayscale (SGL)", "Complex (CSG)", "RGB (U32)", "HSL (U32)", "RGB (U64)", "Grayscale (U16)"]  # Image Type
          w249 = "imaq_file_out"  # Image Name
          n82 = call <vilib>:"IMAQdx Grab2.vi"("error in"=w241, "Image In"=w240, "Session In"=w239) -> ("error out"=w234:errorcluster, "Image Out"=w246:T1, "Session Out"=w236:T2)  [unwired: 5 in, 1 out]
          n83 = call "IMAQ ColorImageToArray"("Image"=w246, "error in (no error)"=w242) -> ("Image Pixels (U32)"=w243:u32[][], "error out"=w247:errorcluster)  [unwired: 2 in, 1 out]
          n84 = call "python.vi"("Image Pixels (U32)"=w243) -> ("error out"=→"Python Error Out":errorcluster, "Array"=w244:u32[][])  [unwired: 9 in]
          n85 = call "IMAQ Create"("Image Name"=w249, "Image Type"=w248) -> ("New Image"=w233:T1)  [unwired: 3 in, 1 out]
          n86 = call "IMAQ ArrayToColorImage"("Image Pixels (U32)"=w244, "Image"=w233, "error in (no error)"=w247) -> ("Image Out"=→"Live view":T1, "error out"=→"IMAQ Err":errorcluster)  [unwired: 2 in]
          "Status" <- "Off/On"
        }
        n87 = call <vilib>:"IMAQdx Close Camera.vi"("error in"=w219, "Session In"=w218) -> ("error out"=w224:errorcluster)  [unwired: 9 in]
        "Camera Status" <- w224
        n88 = call <vilib>:"Add State(s) to Queue__JKI_lib_State_Machine.vi"("State(s) in (\"\")"=w232) -> ("States Out"=w231:string)  [unwired: 14 in]
      }
    }
  }
